vi "decodeStream.vi"(8 "error in (no error)":errorcluster, 9 "beginIndex":i32, 10 "binary stream":u8[](array[numeric]), 11 "tBSONTimestamp in":refnum<class "tBSONTimestamp.lvclass">) -> (0 "error out":errorcluster, 1 "endIndex":i32, 2 "binary stream out":u8[](array[numeric]), 3 "tBSONTimestamp out":refnum<class "tBSONTimestamp.lvclass">)   [LabVIEW 2013, in "BSON.lvlib" / "tBSONTimestamp.lvclass"]
uses:
  tBSONTimestamp.lvclass
  tBSONElement/tBSONElement.lvclass
  setValue.vi
  BSON.lvlib
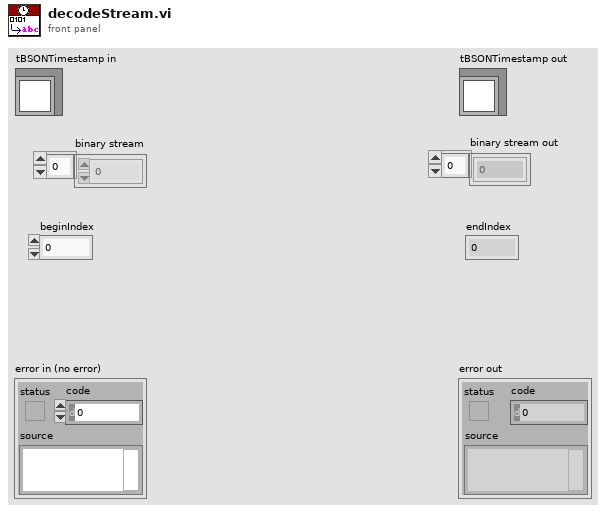
[diagram p1: front panel]
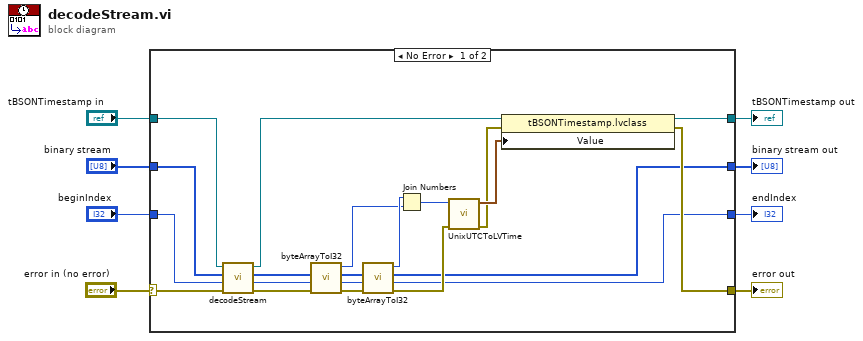
[diagram p0: block diagram]
diagram:
  n1 = case shown="No Error" "error in (no error)" {
    selector: "error in (no error)" -> [w29 w30]
    tunnel: [w23 w30] -> w7
    tunnel: "beginIndex" -> [w26 w31]
    tunnel: "binary stream" -> [w27 w32]
    tunnel: "tBSONTimestamp in" -> [w28 w33]
    tunnel: [w24 w33] -> w3
    tunnel: [w11 w32] -> w2
    tunnel: [w12 w31] -> w1
    frame No Error {
      n2 = call-parent "decodeStream.vi"("error in (no error)"=w29, "beginIndex"=w26, "binary stream"=w27, "tBSONElement in"=w28) -> ("error out"=w22:errorcluster, "endIndex"=w21:i32, "binary stream out"=w20:u8[], "tBSONElement out"=w25:refnum<class "tBSONTimestamp.lvclass">)  [unwired: 4 in]
      n3 = call "byteArrayToI32.vi"("error in (no error)"=w22, "StartIndex"=w21, "ByteArrayIn"=w20) -> ("error out"=w19:errorcluster, "EndIndex"=w18:i32, "ByteArrayOut"=w17:u8[], "I32"=w9:i32)  [unwired: 5 in]
      n4 = call "byteArrayToI32.vi"("error in (no error)"=w19, "StartIndex"=w18, "ByteArrayIn"=w17) -> ("error out"=w15:errorcluster, "EndIndex"=w12:i32, "ByteArrayOut"=w11:u8[], "I32"=w10:i32)  [unwired: 5 in]
      n5 = Join Numbers(hi=w10, lo=w9) -> ((hi.lo)=w16:u64)
      n6 = call "UnixUTCToLVTime.vi"("error in (no error)"=w15, "Unix Time (in milliseconds)"=w16) -> ("error out"=w13:errorcluster, "Local Timestamp"=w14:timestamp)  [unwired: 8 in]
      n7 = property class="tBSONTimestamp.lvclass"(reference=w25, error in=w13, "Value"=w14) -> (reference out=w24:refnum<class "tBSONTimestamp.lvclass">, error out=w23:errorcluster)
    }
    frame Error {
    }
  }
  "error out" <- w7
  "tBSONTimestamp out" <- w3
  "binary stream out" <- w2
  "endIndex" <- w1
